vi "Main.vi"(7 "Name (\"\" to Use UUID)":string="Event CSM") -> ()   [LabVIEW 2020]
uses:
  <userlib>/_NEVSTOP/Communicable State Machine(CSM)/AdvanceAPI/CSM - Break Down Multiple States String.vi
  <userlib>/_NEVSTOP/Communicable State Machine(CSM)/AdvanceAPI/CSM - Compact Multiple States.vi
  <userlib>/_NEVSTOP/Communicable State Machine(CSM)/AdvanceAPI/CSM - Revert Arguments-Safe String.vi
  <userlib>/_NEVSTOP/Communicable State Machine(CSM)/_Shared/Trim Single-line Text.vi
  <userlib>/_NEVSTOP/Communicable State Machine(CSM)/AdvanceAPI/CSM - Make String Arguments Safe.vi
  <userlib>/_NEVSTOP/Communicable State Machine(CSM)/AdvanceAPI/CSM - Keywords.vi
  <userlib>/_NEVSTOP/Communicable State Machine(CSM)/Communicable State Machine.lvlib
  <userlib>/_NEVSTOP/Communicable State Machine(CSM)/_Polymophic/Build No-Reply Asynchronous Message with Arguments.vi
panel:
  in  "Edit Mode?":bool
  in  "Program":bool caption="程序编辑"
  in  "UserManager":bool caption="用户管理"
  in  "TestFilesManager":bool caption="管理文档"
  in  "Help":bool caption="帮助信息"
  in  "Power Square":bool
  in  "SettingMain":bool caption="系统参数"
  in  "DatabaseMain":bool caption="数据查询"
  in  "TesterMain":bool caption="测试序列"
  out "State History":string
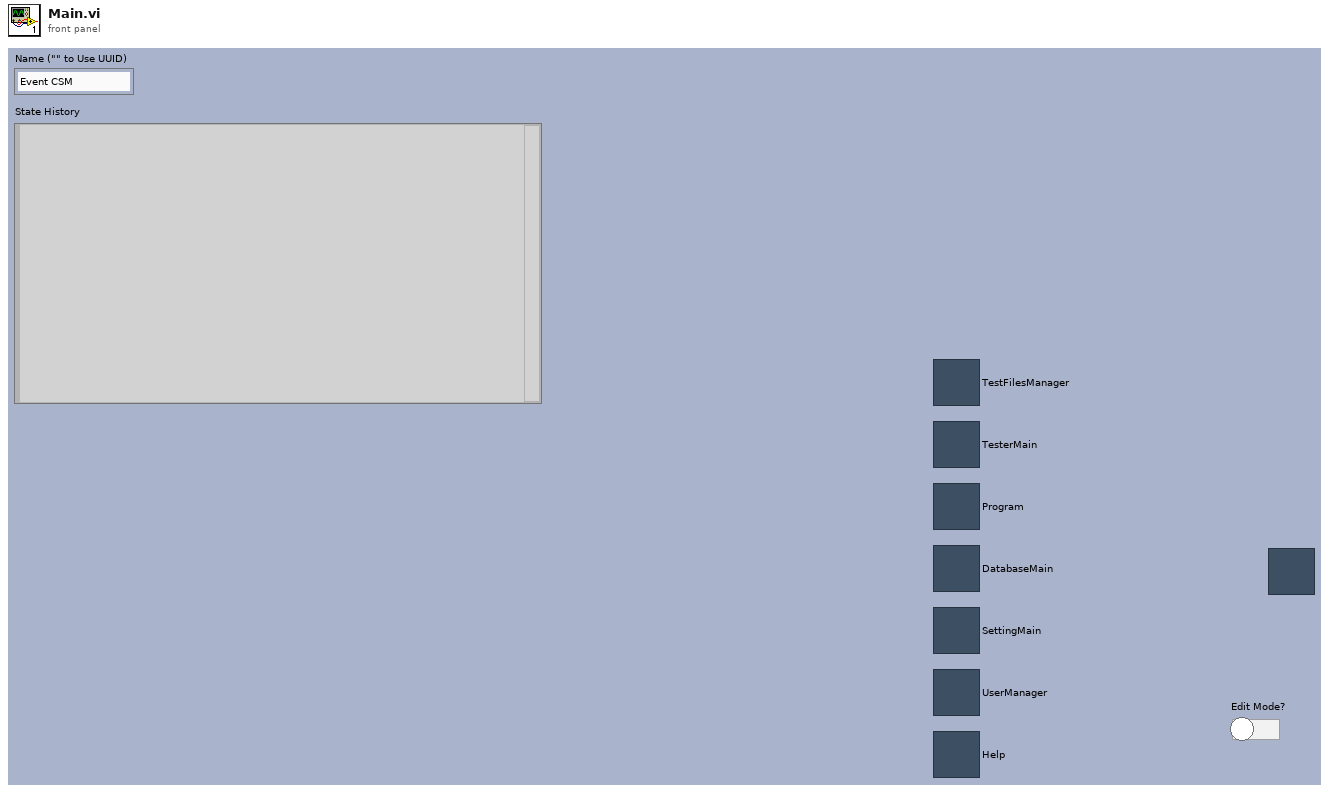
[diagram p1: front panel]
types:
  T1 = enum32{"Invalid", "Standard", "Closed", "Hidden", "Minimized", "Maximized"}
  T2 = enum32{"invalid app kind", "Development System", "Run Time System", "Student Edition", "Embedded LabVIEW", "Evaluation", "Custom"}
  T3 = typedef "Communicable State Machine.lvlib/_CSM_Response Source Message.ctl" = cluster{"‘State":string, "’Arguments":string, "’Error":errorcluster}
  T4 = cluster{"Current VI Reference":refnum<vi>, "Close Panel on Exit?":bool}
  T5 = cluster{"Core":cluster{"Current VI Reference":refnum<vi>, "Close Panel on Exit?":bool}, "Your Boolean data":bool, "Your string data":string}
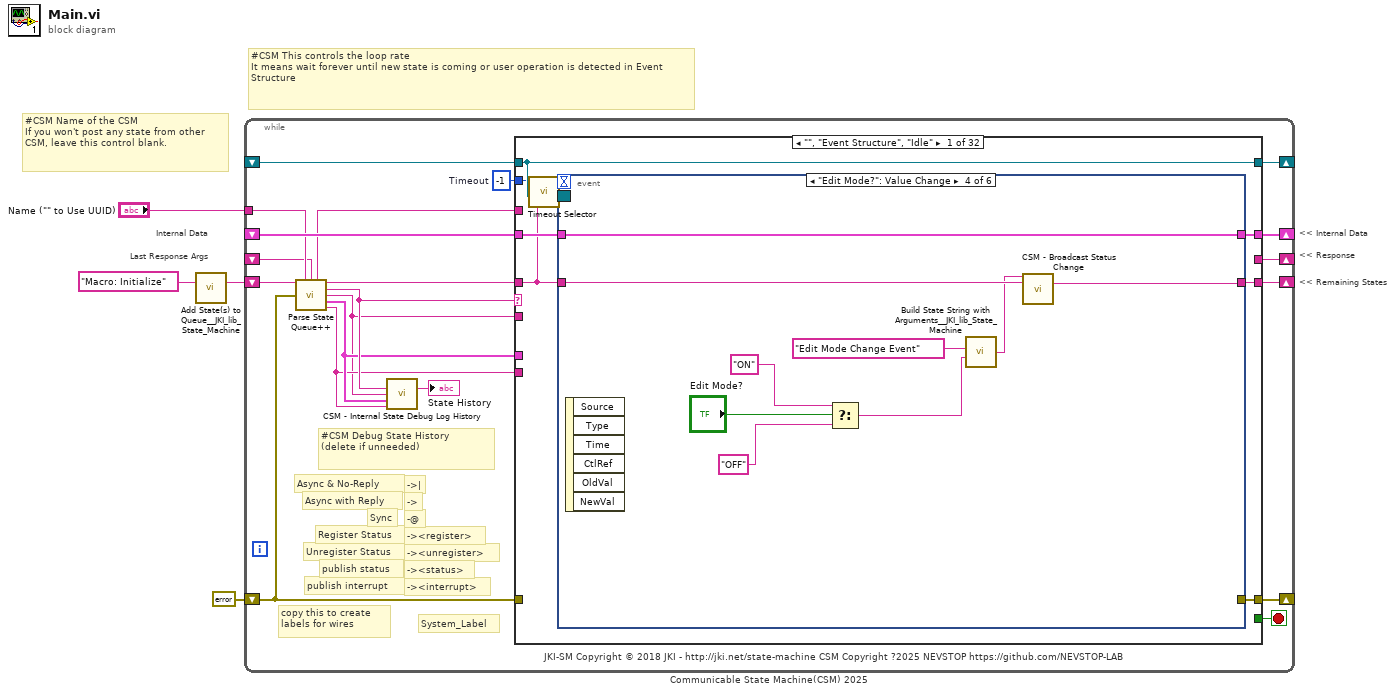
[diagram p0: block diagram]
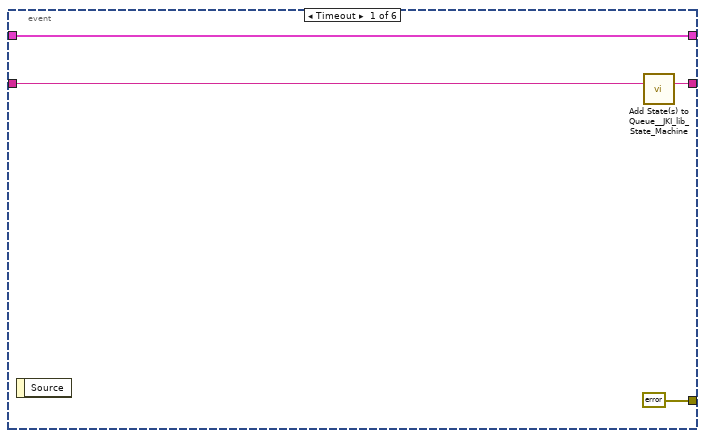
[diagram p2: hidden frame]
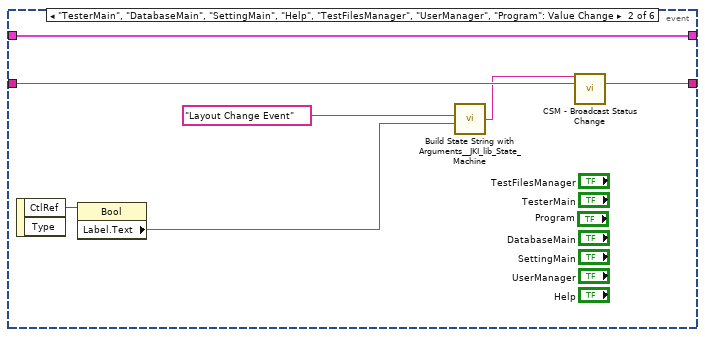
[diagram p3: hidden frame]
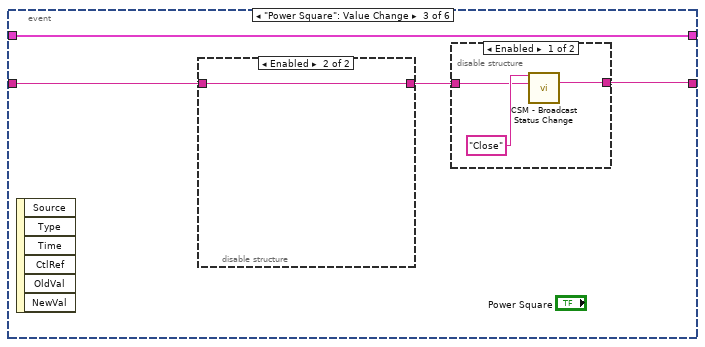
[diagram p4: hidden frame]
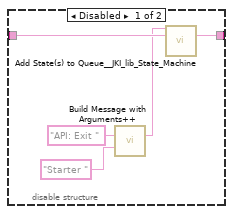
[diagram p5: hidden frame]
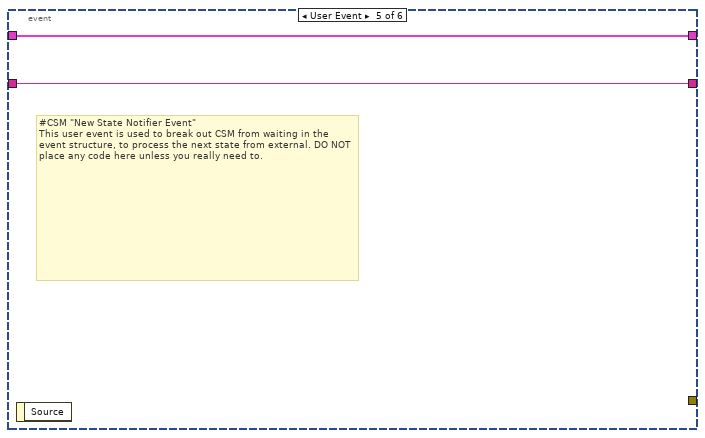
[diagram p7: hidden frame]
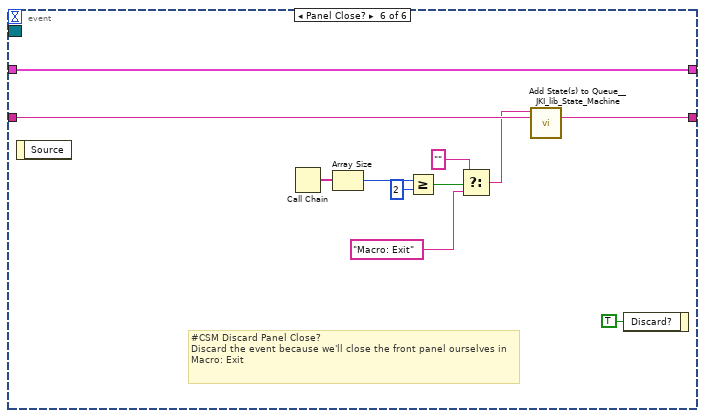
[diagram p8: hidden frame]
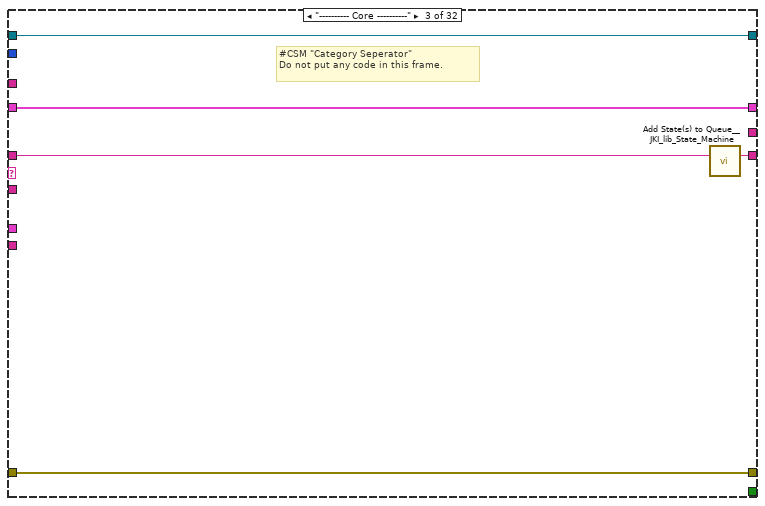
[diagram p10: hidden frame]
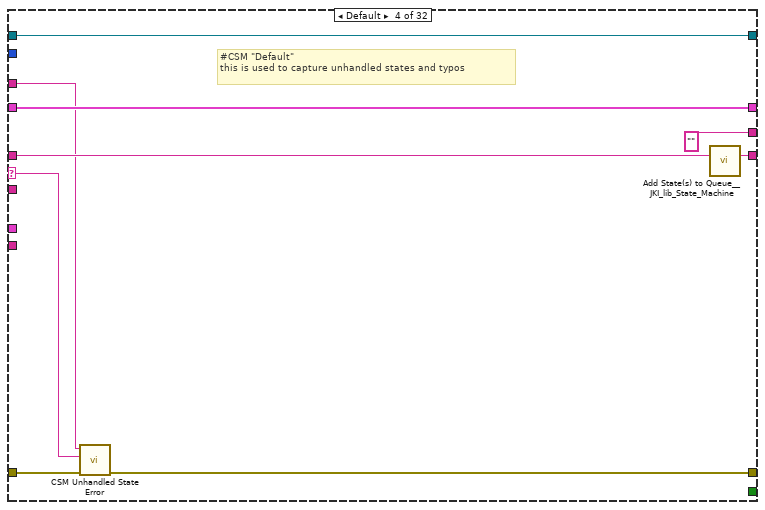
[diagram p11: hidden frame]
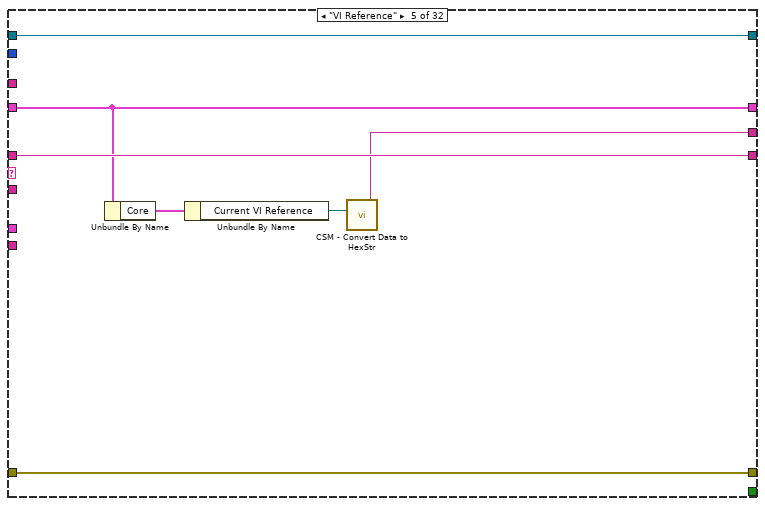
[diagram p12: hidden frame]
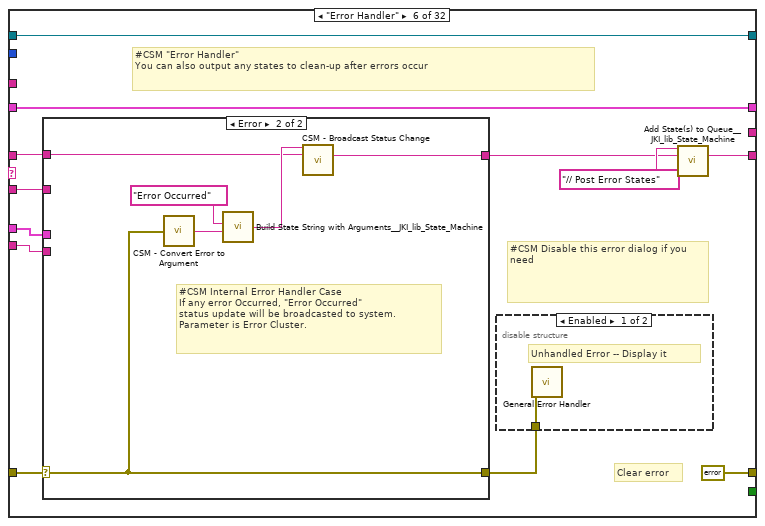
[diagram p13: hidden frame]
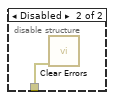
[diagram p14: hidden frame]
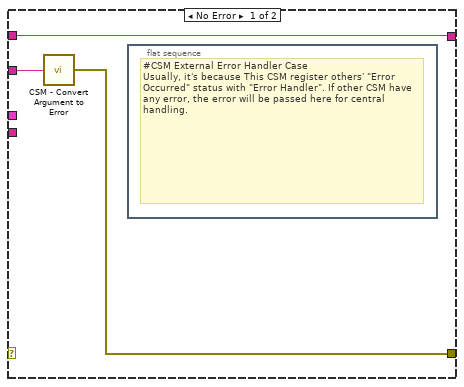
[diagram p15: hidden frame]
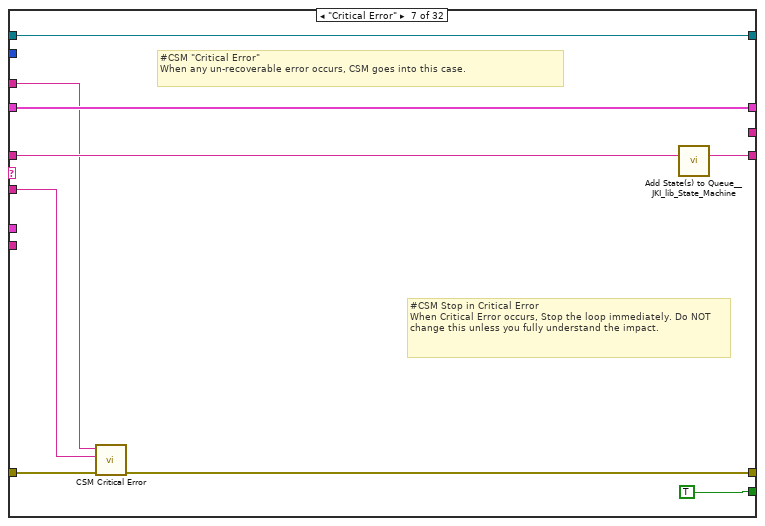
[diagram p16: hidden frame]
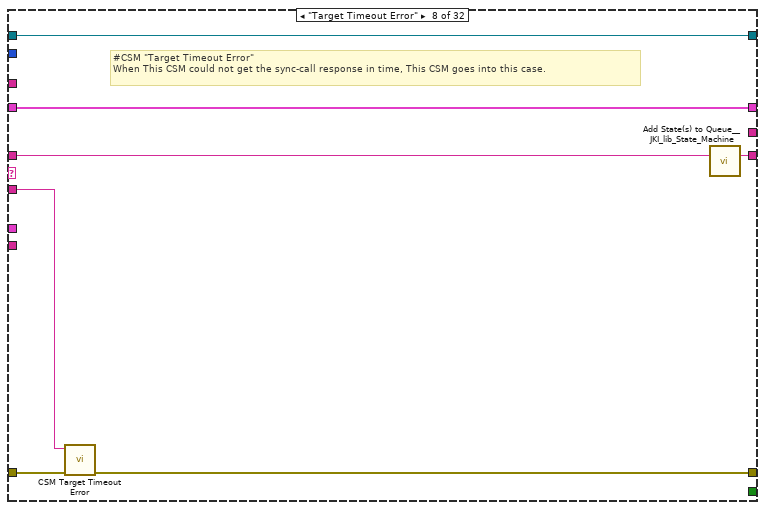
[diagram p17: hidden frame]
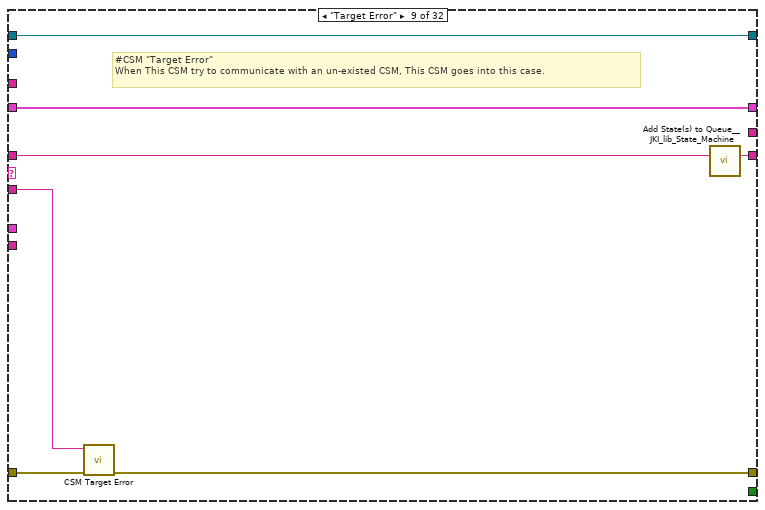
[diagram p18: hidden frame]
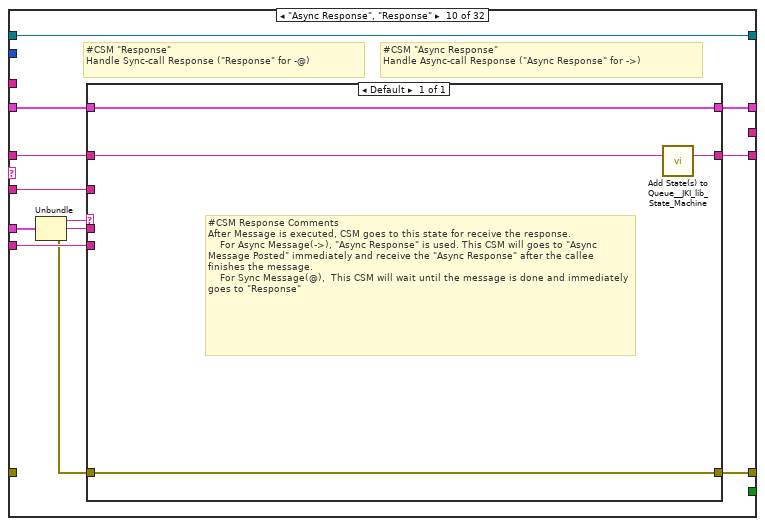
[diagram p19: hidden frame]
diagram:
  # "Last Response Args"
  # "Internal Data"
  # "<< Internal Data"
  # "<< Response"
  # "<< Remaining States"
  # "#CSM Name of the CSM\nIf you won't post any state from other CSM, leave this control blank."
  # "#CSM This controls the loop rate\nIt means wait forever until new state is coming or user operation is detected in Event Structure"
  n1 = call <vilib>:"Add State(s) to Queue__JKI_lib_State_Machine.vi"("State(s) in (\"\")"="Macro: Initialize" ("Init State(\"Macro: Initialize\")")) -> ("States Out"=w1:string)  [unwired: 14 in]
  n2 = while "Communicable State Machine(CSM) 2025" {
    shift-right: [w19] -> _
    shift-left: _ -> [w18]
    shift-right: [w22] -> _
    shift-left: errorcluster {"status"=FALSE, "code"=0, "source"=""} ("error out") -> [w16]
    shift-right: [w21] -> _
    shift-left: w1 -> [w23]
    tunnel: "Name (\"\" to Use UUID)" -> [w12]
    shift-right: [w15] -> _
    shift-left: _ -> [w7]
    shift-right: [w14] -> _
    shift-left: _ -> [w13]
    stop <- w20 stop-if-true
    w17 = -1  # Timeout
    # "#CSM Debug State History\n(delete if unneeded)"
    # "-><interrupt>"
    # "-><status>"
    # "-><unregister>"
    # "-><register>"
    # "-@"
    # "->"
    # "->|"
    # "publish interrupt"
    # "publish status"
    # "Unregister Status"
    # "Register Status"
    # "Sync"
    # "Async with Reply"
    # "Async & No-Reply"
    # "copy this to create labels for wires"
    # "System_Label"
    # "JKI-SM Copyright © 2018 JKI - http://jki.net/state-machine CSM Copyright ?2025 NEVSTOP https://github.com/NEVSTOP-LAB"
    n3 = call <userlib>:"Parse State Queue++.vi"("State Queue"=w23, "Name (\"\" to Use UUID)"=w12, "Response Arguments"=w7, "Previous Error"=w16) -> ("Name Used"=w8:string, "Remaining States"=w24:string, "Current State"=w11:string, "Arguments"=w6:string, "Additional Information"=w10:T3, "Source CSM"=w9:string)  [unwired: 6 in]
    n4 = call <userlib>:"CSM - Internal State Debug Log History.vi"("State"=w11, "Arguments (\"\")"=w6, ">> Response Source Message >>"=w10, "Source (\"\")"=w9) -> ("Debug Log"=→"State History":string)  [unwired: 11 in]
    n5 = case shown="\"\", \"Event Structure\", \"Idle\"" w11 {
      selector: w11 -> [_ _ _ w90 _ _ _ _ _ _ _ _ _ _ _ _ _ _ _ _ _ _ _ _ _ _ _ _ _ _ _ _]
      tunnel: w24 -> [w25 w82 w87 w96 w102 w108 w134 w142 w149 w159 w168 w181 w186 w190 w197 w203 w207 w214 w218 w222 w226 w232 w243 w307 w312 w323 w326 w335 w339 w343 w347 w351]
      tunnel: w6 -> [_ _ _ _ _ w106 w130 w137 w145 w153 _ _ _ _ _ _ _ _ _ _ _ w228 w238 _ _ _ _ _ _ _ _ _]
      tunnel: w18 -> [w31 w81 w84 w94 w101 w114 w135 w140 w147 w157 w167 w175 w184 w188 _ w199 w205 w213 w217 w220 w224 w230 w240 w305 w311 w321 w325 w334 w338 w341 w345 w349]
      tunnel: [w30 _ w85 w88 w103 errorcluster {"status"=FALSE, "code"=0, "source"=""} ("error out") w127 w136 w143 w156 _ _ _ _ _ w200 _ w208 w216 _ _ w229 w241 _ _ _ _ w330 _ _ _ _] -> w22
      tunnel: w16 -> [_ _ w85 w89 w103 w112 w128 w138 w144 _ _ _ _ _ _ _ _ _ _ _ _ _ _ _ _ _ _ w331 _ _ _ _]
      tunnel: [w32 w82 w86 w95 w102 w110 w133 w141 w148 w160 w168 w180 w185 w189 w196 w202 w206 w214 w218 w221 w223 w231 w242 w306 w308 w322 w326 w332 w339 w342 w346 w350] -> w21
      tunnel: [_ _ _ _ _ _ TRUE _ _ _ _ _ TRUE _ _ _ _ _ _ _ _ _ _ _ _ _ _ _ _ _ _ _] -> w20
      tunnel: [w29 w81 w84 w94 w101 w114 w135 w140 w147 w158 w167 w179 w184 w188 w195 w199 w205 w213 w217 w220 w224 w230 w240 w305 w311 w321 w325 w334 w338 w341 w345 w349] -> w19
      tunnel: w17 -> [w27 _ _ _ _ _ _ _ _ _ _ _ _ _ _ _ _ _ _ _ _ _ _ _ _ _ _ _ _ _ _ _]
      tunnel: w9 -> [_ _ _ _ _ w105 _ _ _ w154 _ _ _ _ _ _ _ _ _ _ _ _ _ _ _ _ _ _ _ _ _ _]
      tunnel: w10 -> [_ _ _ _ _ w104 _ _ _ w155 _ _ _ _ _ _ _ _ _ _ _ _ _ _ _ _ _ _ _ _ _ _]
      tunnel: [_ _ _ "" w97 _ _ _ _ _ _ _ _ _ _ _ _ _ _ _ _ _ _ _ _ _ _ _ _ _ _ _] -> w15
      tunnel: [w28 w80 w83 w92 w100 w113 w131 w139 w146 w161 w166 w169 w182 w187 w191 w198 w204 w212 w215 w219 w225 w227 w237 w304 w309 w314 w324 w336 w337 w340 w344 w348] -> w14
      tunnel: w13 -> [w28 w80 w83 w92 w100 w113 w131 w139 w146 w161 w166 w169 w182 w187 w191 w198 w204 _ w215 w219 w225 w227 w237 w304 w309 w314 w324 w336 w337 w340 w344 w348]
      tunnel: w8 -> [_ _ _ w91 _ _ w129 _ _ _ _ _ _ _ _ _ _ w211 _ _ _ _ _ _ _ _ _ w333 _ _ _ _]
      frame "", "Event Structure", "Idle" {
        n6 = call <userlib>:"Timeout Selector.vi"("Remaining States"=w25, "Timeout Expected"=w27) -> ("Timeout"=w26:i32)  [unwired: 5 in]
        n7 = event shown="[3] \"Edit Mode?\": Value Change" {
          selector: w28 -> [_ _ _ _ _ _]
          dyn-events: _ -> [_ _ _ _ _ _]
          timeout: w26 -> [_ _ _ _ _ _]
          tunnel: w25 -> [w36 w42 w45 w65 w67 w79]
          tunnel: [w35 w41 w46 w64 w67 w78] -> w32
          tunnel: w31 -> [w34 w43 w47 w66 w68 w77]
          tunnel: [errorcluster {"status"=FALSE, "code"=0, "source"=""} ("error out") _ _ _ _ _] -> w30
          tunnel: [w34 w43 w47 w66 w68 w77] -> w29
          event Timeout {
            n8 = event-data() -> ()  [unwired: 1 in, 1 out]
            n9 = call <vilib>:"Add State(s) to Queue__JKI_lib_State_Machine.vi"("State(s) in (\"\")"=w36) -> ("States Out"=w35:string)  [unwired: 14 in]
          }
          event "TesterMain", "DatabaseMain", "SettingMain", "Help", "TestFilesManager", "UserManager", "Program": Value Change {
            n10 = event-data() -> ("CtlRef"=w39:refnum<vi>)  [unwired: 1 in, 1 out]
            n11 = property class="Bool"(reference=w39) -> ("Label.Text"=w38:string)  [unwired: 1 in, 2 out]
            n12 = call <vilib>:"Build State String with Arguments__JKI_lib_State_Machine.vi"("Arguments (\"\")"=w38, "State"="Layout Change Event") -> ("State with Arguments"=w40:string)  [unwired: 4 in]
            n13 = call <userlib>:"CSM - Broadcast Status Change.vi"("Status With Arguments"=w40, "State Queue"=w42) -> ("Remaining States"=w41:string)  [unwired: 13 in]
          }
          event "Power Square": Value Change {
            n14 = event-data() -> ()  [unwired: 1 in, 6 out]
            n15 = disable-structure shown="Enabled" {
              disable-tunnel: w45 -> [w52 w53]
              disable-tunnel: [w51 w53] -> w44
              frame Disabled {
                n16 = call-poly <userlib>:"Build Message with Arguments++.vi"("State With Arguments"="API: Exit ", "Target Module (\"\")"="Starter " ("State With Arguments")) -> ("CSM Message String"=w48:string)  [unwired: 13 in]
                n17 = call <vilib>:"Add State(s) to Queue__JKI_lib_State_Machine.vi"("State(s) in Front (\"\")"=w48, "State(s) in (\"\")"=w52) -> ("States Out"=w51:string)  [unwired: 13 in]
              }
              frame Enabled {
              }
            }
            n18 = disable-structure shown="Enabled" {
              disable-tunnel: [w55 w57] -> w46
              disable-tunnel: w44 -> [w54 w57]
              frame Enabled {
                n19 = call <userlib>:"CSM - Broadcast Status Change.vi"("Status With Arguments"="Close" ("State"), "State Queue"=w54) -> ("Remaining States"=w55:string)  [unwired: 13 in]
              }
              frame Disabled {
              }
            }
          }
          event "Edit Mode?": Value Change {
            n20 = event-data() -> ()  [unwired: 1 in, 6 out]
            n21 = Select(t="ON" ("Arguments (\"\")"), s="Edit Mode?", f="OFF" ("Arguments (\"\")")) -> (s? t:f=w61:string)
            n22 = call <vilib>:"Build State String with Arguments__JKI_lib_State_Machine.vi"("Arguments (\"\")"=w61, "State"="Edit Mode Change Event") -> ("State with Arguments"=w59:string)  [unwired: 4 in]
            n23 = call <userlib>:"CSM - Broadcast Status Change.vi"("Status With Arguments"=w59, "State Queue"=w65) -> ("Remaining States"=w64:string)  [unwired: 13 in]
          }
          event User Event {
            # "#CSM \"New State Notifier Event\"\nThis user event is used to break out CSM from waiting in the event structure, to process the next state from external. DO NOT place any code here unless you really need to."
            n24 = event-data() -> ()  [unwired: 1 in, 1 out]
          }
          event Panel Close? {
            # "#CSM Discard Panel Close?\nDiscard the event because we'll close the front panel ourselves in Macro: Exit"
            n25 = event-data() -> ()  [unwired: 1 in, 1 out]
            n26 = Call Chain() -> (call chain=w69:string[])
            n27 = Array Size(array=w69) -> (size(s)=w75:i32)
            n28 = Greater Or Equal?(x=w75, y=2) -> (x >= y?=w73:bool)
            n29 = Select(t="", s=w73, f="Macro: Exit") -> (s? t:f=w70:string)
            n30 = call <vilib>:"Add State(s) to Queue__JKI_lib_State_Machine.vi"("State(s) in Front (\"\")"=w70, "State(s) in (\"\")"=w79) -> ("States Out"=w78:string)  [unwired: 13 in]
            n31 = event-data("Discard?"=TRUE) -> ()  [unwired: 1 in, 1 out]
          }
        }
      }
      frame "CSM Documentation" {
        # "#CSM State Syntax\n\n// Comment line, all text to the right of “//” will be ignored\n// Local Message Example\nDoSth: DoA >> Arguments\n\n// Sync Call Example\nAPI: xxxx >> Arguments -@ TargetModule\n\n// Async Call Example\nAPI: xxxx >> Arguments -> TargetModule\n\n// Async Call without Reply Example\nAPI: xxxx >> Arguments ->| TargetModule\n\n// Broadcast normal status:\nStatus >> StatusArguments  -><status>\n\n// Broadcast Interrupt status:\nInterrupt >> StatusArguments  -><interrupt>\n\n// Register Source Module's status to Handler Module\nStatus@Source Module >> Handler Module@Handler Module -><register>\n\n// Unegister Source Module's status\nStatus@Source Module >> Handler Module -><unregister>"
        # "#CSM README FIRST\n\nCommunicable State Machine(CSM) is a LabVIEW application framework that builds upon JKI State Machine(JKISM). It follows the pattern of JKISM and extends the keywords to describe message communication between modules, including concepts such as Sync-Message, Async-Message, Subscription/Unsubscription of status - essential elements for creating reusable code modules. For more information, please visit the CSM wiki: https://nevstop-lab.github.io/CSM-Wiki/\n\nFor instructions on JKI State Machine, visit: \n    http://jki.net/state-machine/\nFor information about CSM, visit: \n    https://github.com/NEVSTOP-LAB"
        # "#CSM \"Documentation\"\nCase for holding CSM Documenation"
      }
      frame "---------- Core ----------" {
        # "#CSM \"Category Seperator\"\nDo not put any code in this frame."
        n32 = call <vilib>:"Add State(s) to Queue__JKI_lib_State_Machine.vi"("State(s) in (\"\")"=w87) -> ("States Out"=w86:string)  [unwired: 14 in]
      }
      frame Default {
        # "#CSM \"Default\"\nthis is used to capture unhandled states and typos"
        n33 = call <userlib>:"CSM Unhandled State Error.vi"("error in (no error)"=w89, "Undefined State"=w90, "CSM Name"=w91) -> ("error out"=w88:errorcluster)  [unwired: 8 in]
        n34 = call <vilib>:"Add State(s) to Queue__JKI_lib_State_Machine.vi"("State(s) in (\"\")"=w96) -> ("States Out"=w95:string)  [unwired: 14 in]
      }
      frame "VI Reference" {
        n35 = Unbundle By Name(w101) -> ("Core"=w99:T4)
        n36 = Unbundle By Name(w99) -> ("Current VI Reference"=w98:refnum<vi>)
        n37 = call <userlib>:"CSM - Convert Data to HexStr.vi"("Variant"=w98) -> ("HEX String (0-9,A-F)"=w97:string)  [unwired: 8 in]
      }
      frame "Error Handler" {
        # "#CSM Disable this error dialog if you need"
        # "#CSM \"Error Handler\"\nYou can also output any states to clean-up after errors occur"
        # "Clear error"
        n38 = case shown="Error" w112 {
          selector: w112 -> [_ w121]
          tunnel: [w119 w123] -> w109
          tunnel: w108 -> [w119 w122]
          tunnel: [w118 w121] -> w107
          tunnel: w106 -> [w120 _]
          tunnel: w105 -> [_ _]
          tunnel: w104 -> [_ _]
          frame No Error {
            n39 = call <userlib>:"CSM - Convert Argument to Error.vi"("Argument"=w120) -> ("Error"=w118:errorcluster)  [unwired: 4 in]
            n40 = flat-sequence {
              frame #0 {
                # "#CSM External Error Handler Case\nUsually, it's because This CSM register others' \"Error Occurred\" status with \"Error Handler\". If other CSM have any error, the error will be passed here for central handling."
              }
            }
          }
          frame Error {
            # "#CSM Internal Error Handler Case \nIf any error Occurred, \"Error Occurred\" \nstatus update will be broadcasted to system.\nParameter is Error Cluster."
            n41 = call <userlib>:"CSM - Convert Error to Argument.vi"("Error"=w121) -> ("Argument"=w125:string)  [unwired: 4 in]
            n42 = call <vilib>:"Build State String with Arguments__JKI_lib_State_Machine.vi"("Arguments (\"\")"=w125, "State"="Error Occurred" ("Status with Arguments")) -> ("State with Arguments"=w124:string)  [unwired: 4 in]
            n43 = call <userlib>:"CSM - Broadcast Status Change.vi"("Status With Arguments"=w124, "State Queue"=w122) -> ("Remaining States"=w123:string)  [unwired: 13 in]
          }
        }
        n44 = disable-structure shown="Enabled" {
          disable-tunnel: w107 -> [w116 w117]
          frame Enabled {
            # "Unhandled Error -- Display it"
            n45 = call <vilib>:"General Error Handler.vi"("error in (no error)"=w116) -> ()  [unwired: 10 in, 5 out]
          }
          frame Disabled {
            n46 = call <vilib>:"Clear Errors.vi"("error in (no error)"=w117) -> ()  [unwired: 5 in, 2 out]
          }
        }
        n47 = call <vilib>:"Add State(s) to Queue__JKI_lib_State_Machine.vi"("State(s) in Front (\"\")"="// Post Error States", "State(s) in (\"\")"=w109) -> ("States Out"=w110:string)  [unwired: 13 in]
      }
      frame "Critical Error" {
        # "#CSM \"Critical Error\"\nWhen any un-recoverable error occurs, CSM goes into this case."
        # "#CSM Stop in Critical Error\nWhen Critical Error occurs, Stop the loop immediately. Do NOT change this unless you fully understand the impact."
        n48 = call <userlib>:"CSM Critical Error.vi"("error in (no error)"=w128, "Arugments (As Reason)"=w130, "CSM Name"=w129) -> ("error out"=w127:errorcluster)  [unwired: 8 in]
        n49 = call <vilib>:"Add State(s) to Queue__JKI_lib_State_Machine.vi"("State(s) in (\"\")"=w134) -> ("States Out"=w133:string)  [unwired: 14 in]
      }
      frame "Target Timeout Error" {
        # "#CSM \"Target Timeout Error\"\nWhen This CSM could not get the sync-call response in time, This CSM goes into this case."
        n50 = call <userlib>:"CSM Target Timeout Error.vi"("error in (no error)"=w138, "Arguments (As CSM Name)"=w137) -> ("error out"=w136:errorcluster)  [unwired: 9 in]
        n51 = call <vilib>:"Add State(s) to Queue__JKI_lib_State_Machine.vi"("State(s) in (\"\")"=w142) -> ("States Out"=w141:string)  [unwired: 14 in]
      }
      frame "Target Error" {
        # "#CSM \"Target Error\"\nWhen This CSM try to communicate with an un-existed CSM, This CSM goes into this case."
        n52 = call <userlib>:"CSM Target Error.vi"("error in (no error)"=w144, "Arguments (As CSM Name)"=w145) -> ("error out"=w143:errorcluster)  [unwired: 9 in]
        n53 = call <vilib>:"Add State(s) to Queue__JKI_lib_State_Machine.vi"("State(s) in (\"\")"=w149) -> ("States Out"=w148:string)  [unwired: 14 in]
      }
      frame "Async Response", "Response" {
        # "#CSM \"Async Response\"\nHandle Async-call Response (\"Async Response\" for ->)"
        # "#CSM \"Response\"\nHandle Sync-call Response (\"Response\" for -@)"
        n54 = Unbundle(w155) -> ("‘State"=w152:string, "’Arguments"=w151:string, "’Error"=w150:errorcluster)
        n55 = case shown="Default" w152 {
          tunnel: [w162] -> w160
          tunnel: w159 -> [w163]
          tunnel: [w165] -> w158
          tunnel: w157 -> [w165]
          tunnel: [w164] -> w156
          tunnel: w150 -> [w164]
          tunnel: w154 -> [_]
          tunnel: w153 -> [_]
          tunnel: w151 -> [_]
          frame Default {
            # "#CSM Response Comments\nAfter Message is executed, CSM goes to this state for receive the response.\n    For Async Message(->), \"Async Response\" is used. This CSM will goes to \"Async Message Posted\" immediately and receive the \"Async Response\" after the callee finishes the message.\n    For Sync Message(@),  This CSM will wait until the message is done and immediately goes to \"Response\""
            n56 = call <vilib>:"Add State(s) to Queue__JKI_lib_State_Machine.vi"("State(s) in (\"\")"=w163) -> ("States Out"=w162:string)  [unwired: 14 in]
          }
        }
      }
      frame "Async Message Posted" {
        # "#CSM \"Async Message Posted\"\nAfter Async Message is posted (-> or ->| ), CSM goes to this state for post-action.\nYou can use Argument - State to tell which Async Message is called."
      }
      frame "Initialize Core Data" {
        # "#CSM \"Initialize Core Data\"\nThis is used to determine panel behavior on exit"
        # "originally closed?"
        # "exe?"
        # "If panel starts closed or is an EXE, then close it when we exit"
        n57 = property class="VI"() -> ("FP.State"=w172:T1)  [unwired: 2 in, 2 out]
        n58 = property class="App"() -> ("App.Kind"=w178:T2)  [unwired: 2 in, 2 out]
        n59 = control-ref of="Current VI Reference"() -> (w173:refnum<vi>)
        n60 = Equal?(x=w172, y=T1."Closed" ("Front Panel Window:State")) -> (x = y?=w170:bool)
        n61 = Equal?(x=w178, y=T2."Run Time System" ("Application:Kind")) -> (x = y?=w176:bool)
        n62 = Or(x=w170, y=w176) -> (x .or. y?=w174:bool)
        n63 = Bundle By Name(cluster=w175, "Core.Current VI Reference"=w173, "Core.Close Panel on Exit?"=w174) -> (w179:T5)
        n64 = call <vilib>:"Add State(s) to Queue__JKI_lib_State_Machine.vi"("State(s) in (\"\")"=w181) -> ("States Out"=w180:string)  [unwired: 14 in]
      }
      frame "Exit" {
        # "#CSM \"Exit\"\nCase for exiting the loop. No errors that occur here will be handled."
        n65 = call <vilib>:"Add State(s) to Queue__JKI_lib_State_Machine.vi"("State(s) in (\"\")"=w186) -> ("States Out"=w185:string)  [unwired: 14 in]
      }
      frame "---------- Data ----------" {
        # "#CSM \"Category Seperator\"\nDo not put any code in this frame."
        n66 = call <vilib>:"Add State(s) to Queue__JKI_lib_State_Machine.vi"("State(s) in (\"\")"=w190) -> ("States Out"=w189:string)  [unwired: 14 in]
      }
      frame "Data: Initialize" {
        w192 = T4 {"Current VI Reference"=refnum, "Close Panel on Exit?"=FALSE}  # Core
        w194 = TRUE  # Your Boolean data
        w193 = ""  # Your string data
        # "#CSM  do not delete - used by framework"
        # "#CSM Expand Bundle to add new data elements to shift register data."
        # "#CSM Add new data here."
        # "#CSM Data names and types of shift register data are defined by this bundle."
        # "#CSM \"Data: Initialize\"\nInitialize the shift-register data, here.\n(data names are defined by what you wire into the bundle function)"
        n67 = Bundle("Core"=w192, "Your Boolean data"=w194, "Your string data"=w193) -> (w195:T5)  [unwired: 1 in]
        n68 = call <vilib>:"Add State(s) to Queue__JKI_lib_State_Machine.vi"("State(s) in (\"\")"=w197) -> ("States Out"=w196:string)  [unwired: 14 in]
      }
      frame "Data: Cleanup" {
        # "#CSM \"Data: Cleanup\"\nCleanup any data and references, here.\n(this is called automatically, by the Macro: Exit)"
        n69 = Unbundle By Name(w199) -> ("Core.Current VI Reference"=w201:refnum<vi>)
        n70 = Close Reference(reference=w201) -> (error out=w200:errorcluster)  [unwired: 1 in]
        n71 = call <vilib>:"Add State(s) to Queue__JKI_lib_State_Machine.vi"("State(s) in (\"\")"=w203) -> ("States Out"=w202:string)  [unwired: 14 in]
      }
      frame "---------- Events ----------" {
        # "#CSM \"Category Seperator\"\nDo not put any code in this frame."
        n72 = call <vilib>:"Add State(s) to Queue__JKI_lib_State_Machine.vi"("State(s) in (\"\")"=w207) -> ("States Out"=w206:string)  [unwired: 14 in]
      }
      frame "Events: Register" {
        # "#CSM \"Events: Register\"\nRegister user event. New Message Event is registered to break CSM waiting in event structure by default."
        # "#CSM Register New Message Event\nRegister message event to break Waiting in Event structure."
        n73 = call <userlib>:"CSM - Get New State Notifier Event.vi"("Name (\"\" to Use UUID)"=w211) -> ("error out"=w209:errorcluster, "New State Notifier Event"=w210:refnum<user-event>)  [unwired: 9 in]
        n74 = register-events(error in=w209, w210) -> (reference out=w212:refnum<event-registration>, error out=w208:errorcluster)  [unwired: 1 in]
      }
      frame "Events: Unregister" {
        # "#CSM \"Events: Unregister\"\nUnregister user event."
        n75 = Unregister For Events(event registration refnum=w215) -> (error out=w216:errorcluster)  [unwired: 1 in]
      }
      frame "---------- UI ----------" {
        # "#CSM \"Category Seperator\"\nDo not put any code in this frame."
        n76 = call <vilib>:"Add State(s) to Queue__JKI_lib_State_Machine.vi"("State(s) in (\"\")"=w222) -> ("States Out"=w221:string)  [unwired: 14 in]
      }
      frame "UI: Initialize" {
        n77 = call <vilib>:"Add State(s) to Queue__JKI_lib_State_Machine.vi"("State(s) in (\"\")"=w226) -> ("States Out"=w223:string)  [unwired: 14 in]
      }
      frame "UI: Cursor Set" {
        # "Argument"
        # "#CSM \"UI: Cursor Set\"\nSet and Unset Cursor Busy.\n(Usage: \"UI: Cursor Set >> Busy|Idle\")"
        n78 = disable-structure shown="TARGET_TYPE!=Windows" {
          disable-tunnel: [w234 _] -> w229
          disable-tunnel: w228 -> [w233 _]
          frame condition #0 (active) {
            n79 = case shown="\"Idle\", Default" w233 {
              tunnel: [w235 w236] -> w234
              frame "Idle", Default {
                n80 = call <vilib>:"Unset Busy.vi"() -> ("error out"=w235:errorcluster)  [unwired: 11 in]
              }
              frame "Busy" {
                n81 = call <vilib>:"Set Busy.vi"() -> ("error out"=w236:errorcluster)  [unwired: 10 in, 1 out]
              }
            }
          }
          frame condition #1 {
          }
        }
        n82 = call <vilib>:"Add State(s) to Queue__JKI_lib_State_Machine.vi"("State(s) in (\"\")"=w232) -> ("States Out"=w231:string)  [unwired: 14 in]
      }
      frame "UI: Front Panel State" {
        # "Argument"
        # "#CSM \"UI: Front Panel State\"\nSet Front Panel Open or Closed\n(Usage: \"UI: Front Panel State >> Open|Close\")"
        n83 = Unbundle By Name(w240) -> ("Core.Current VI Reference"=w239:refnum<vi>)
        n84 = case shown="\"Open\", \"Standard\", Default" w238 {
          tunnel: [w250 w263 w274 w286 w298] -> w241
          tunnel: w239 -> [w249 w261 w273 w285 w297]
          frame "Open", "Standard", Default {
            w244 = T1."Standard" ("State")
            n85 = property class="VI"(reference=w249) -> (reference out=w247:refnum<vi>, error out=w248:errorcluster, "FP.State"=w246:T1)  [unwired: 1 in]
            n86 = Not Equal?(x=w246, y=w244) -> (x != y?=w245:bool)
            n87 = case shown="True" w245 {
              tunnel: [w254 w256] -> w250
              tunnel: w248 -> [w253 w256]
              tunnel: w247 -> [w252 _]
              tunnel: w244 -> [w251 _]
              frame True {
                n88 = invoke class="VI" method="FP.Open"(reference=w252, error in=w253, "Activate"=TRUE, "State"=w251) -> (error out=w254:errorcluster)  [unwired: 1 in, 4 out]
              }
              frame False {
              }
            }
          }
          frame "Close", "Closed" {
            n89 = property class="VI"(reference=w261) -> (reference out=w260:refnum<vi>, error out=w262:errorcluster, "FP.State"=w258:T1)  [unwired: 1 in]
            n90 = Not Equal?(x=w258, y=T1."Closed" ("Front Panel Window:State")) -> (x != y?=w257:bool)
            n91 = case shown="True" w257 {
              tunnel: [w264 w267] -> w263
              tunnel: w262 -> [w264 w266]
              tunnel: w260 -> [_ w265]
              frame False {
              }
              frame True {
                n92 = invoke class="VI" method="FP.Close"(reference=w265, error in=w266) -> (error out=w267:errorcluster)  [unwired: 1 in, 2 out]
              }
            }
          }
          frame "Hidden", "Hide" {
            w268 = T1."Hidden" ("State")
            n93 = property class="VI"(reference=w273) -> (reference out=w271:refnum<vi>, error out=w272:errorcluster, "FP.State"=w270:T1)  [unwired: 1 in]
            n94 = Not Equal?(x=w270, y=w268) -> (x != y?=w269:bool)
            n95 = case shown="True" w269 {
              tunnel: [w278 w279] -> w274
              tunnel: w272 -> [w277 w279]
              tunnel: w271 -> [w276 _]
              tunnel: w268 -> [w275 _]
              frame True {
                n96 = invoke class="VI" method="FP.Open"(reference=w276, error in=w277, "State"=w275) -> (error out=w278:errorcluster)  [unwired: 2 in, 4 out]
              }
              frame False {
              }
            }
          }
          frame "Minimize", "Minimized" {
            w280 = T1."Minimized" ("State")
            n97 = property class="VI"(reference=w285) -> (reference out=w283:refnum<vi>, error out=w284:errorcluster, "FP.State"=w282:T1)  [unwired: 1 in]
            n98 = Not Equal?(x=w282, y=w280) -> (x != y?=w281:bool)
            n99 = case shown="False" w281 {
              tunnel: [w290 w291] -> w286
              tunnel: w284 -> [w289 w291]
              tunnel: w283 -> [w288 _]
              tunnel: w280 -> [w287 _]
              frame True {
                n100 = invoke class="VI" method="FP.Open"(reference=w288, error in=w289, "State"=w287) -> (error out=w290:errorcluster)  [unwired: 2 in, 4 out]
              }
              frame False {
              }
            }
          }
          frame "Maximize", "Maximized" {
            w292 = T1."Maximized" ("State")
            n101 = property class="VI"(reference=w297) -> (reference out=w295:refnum<vi>, error out=w296:errorcluster, "FP.State"=w294:T1)  [unwired: 1 in]
            n102 = Not Equal?(x=w294, y=w292) -> (x != y?=w293:bool)
            n103 = case shown="True" w293 {
              tunnel: [w302 w303] -> w298
              tunnel: w296 -> [w301 w303]
              tunnel: w295 -> [w300 _]
              tunnel: w292 -> [w299 _]
              frame True {
                n104 = invoke class="VI" method="FP.Open"(reference=w300, error in=w301, "State"=w299) -> (error out=w302:errorcluster)  [unwired: 2 in, 4 out]
              }
              frame False {
              }
            }
          }
        }
        n105 = call <vilib>:"Add State(s) to Queue__JKI_lib_State_Machine.vi"("State(s) in (\"\")"=w243) -> ("States Out"=w242:string)  [unwired: 14 in]
      }
      frame "---------- Macro ----------" {
        # "#CSM \"Category Seperator\"\nDo not put any code in this frame."
        n106 = call <vilib>:"Add State(s) to Queue__JKI_lib_State_Machine.vi"("State(s) in (\"\")"=w307) -> ("States Out"=w306:string)  [unwired: 14 in]
      }
      frame "Macro: Initialize" {
        w310 = "Data: Initialize\nInitialize Core Data\nEvents: Register\nUI: Initialize\nAPI: Update View\n//UI: Front Panel State >> Open"  # Data: Initialize Initialize Core Data Events: Register UI: Initialize API: Update View //UI: Front Panel State >> Open
        # "#CSM \"Macro: Initialize\"\nInitialization Macro (This is called once, when the VI starts)"
        n107 = call <vilib>:"Add State(s) to Queue__JKI_lib_State_Machine.vi"("State(s) in Front (\"\")"=w310, "State(s) in (\"\")"=w312) -> ("States Out"=w308:string)  [unwired: 13 in]
      }
      frame "Macro: Exit" {
        # "#CSM \"Macro: Exit\"\nExit Macro (This is called once, when the VI exits)"
        n108 = Unbundle By Name(w321) -> ("Core.Close Panel on Exit?"=w320:bool)
        n109 = Select(t="UI: Front Panel State >> Close", s=w320, f="") -> (s? t:f=w317:string)
        n110 = call <vilib>:"Add State(s) to Queue__JKI_lib_State_Machine.vi"("State(s) in Front (\"\")"="//Exit Sub-Modules ", "State(s) in (\"\")"=w317, "State(s) at Back (\"\")"="Data: Cleanup\nEvents: Unregister\nExit") -> ("States Out"=w315:string)  [unwired: 12 in]
        n111 = call <vilib>:"Add State(s) to Queue__JKI_lib_State_Machine.vi"("State(s) in Front (\"\")"=w315, "State(s) in (\"\")"=w323) -> ("States Out"=w322:string)  [unwired: 13 in]
      }
      frame "---------- API ----------" {
        # "#CSM \"Category Seperator\"\nDo not put any code in this frame."
      }
      frame "API: Update View" {
        n112 = Unbundle By Name(w334) -> ("Core.Current VI Reference"=w329:refnum<vi>)
        n113 = property on="Pane" class="Pane"() -> ("Height"=w328:u32, "Width"=w327:u32)  [unwired: 2 in, 2 out]
        n114 = call "Update View Event.vi"("VIRef"=w329, "Name"=w333, "error in (no error)"=w331, "Wight"=w327, "Height"=w328, "States Out"=w335) -> ("error out"=w330:errorcluster, "Remaining States"=w332:string)  [unwired: 4 in]
      }
      frame "API: API2" {
        # "#CSM API Example\nCopy/Rename this case for your own API"
      }
      frame "---------- Action ----------" {
        # "#CSM \"Category Seperator\"\nDo not put any code in this frame."
        n115 = call <vilib>:"Add State(s) to Queue__JKI_lib_State_Machine.vi"("State(s) in (\"\")"=w343) -> ("States Out"=w342:string)  [unwired: 14 in]
      }
      frame "Action: action1" {
        # "#CSM \"Internal State\"\nThis category is used for holding internal states"
        n116 = call <vilib>:"Add State(s) to Queue__JKI_lib_State_Machine.vi"("State(s) in (\"\")"=w347) -> ("States Out"=w346:string)  [unwired: 14 in]
      }
      frame "Action: action2" {
        # "#CSM \"Internal State\"\nThis category is used for holding internal states"
        n117 = call <vilib>:"Add State(s) to Queue__JKI_lib_State_Machine.vi"("State(s) in (\"\")"=w351) -> ("States Out"=w350:string)  [unwired: 14 in]
      }
    }
  }
